vi "Test_Moter_Connect.vi"() -> ()   [LabVIEW 2016, in "Motor Base.lvlib"]
uses:
  Motor Base.lvlib
panel:
  out "shared variable refnum out":refnum<k21>
  out "timestamp":timestamp
  out "Transmit PDO mapping 1-Modes of operation display":i8
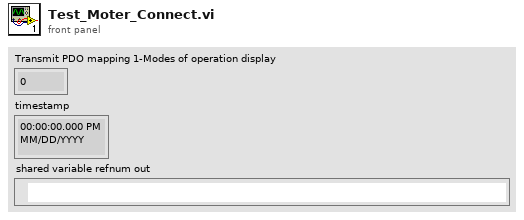
[diagram p1: front panel]
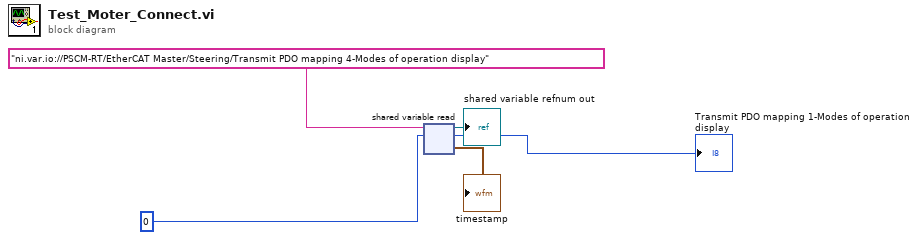
[diagram p0: block diagram]
diagram:
  n1 = shared-variable-read("ni.var.io://PSCM-RT/EtherCAT Master/Steering/Transmit PDO mapping 4-Modes of operation display", i8 0 ("Transmit PDO mapping 1-Modes of operation display 2")) -> (→"shared variable refnum out":refnum<k21>, →"Transmit PDO mapping 1-Modes of operation display":i8, →"timestamp":timestamp)  [unwired: 1 in, 1 out]
